vi "SIM_Drive_ODOM_BEGIN.vi"(8 "error in (no error)":errorcluster, 9 "Initial Pose":T3 {"ROTATION"."SIN" format="%13.4f"; "ROTATION"."COS" format="%13.4f"; "ROTATION"."VALUE" format="%13.4f"; "TRANSLATION"."Y" format="%14.3f"; "TRANSLATION"."X" format="%14.3f"}, 10 "Initial Gyro Angle":T2 {"SIN" format="%13.4f"; "COS" format="%13.4f"; "VALUE" format="%13.4f"}, 11 "Module Positions":T1[](array[typedef]) {"Angle"."SIN" format="%13.4f"; "Angle"."COS" format="%13.4f"; "Angle"."VALUE" format="%13.4f"}) -> (0 "error out":errorcluster)   [LabVIEW 2023]
uses:
  <vilib>/Rock Robotics/WPI/ThirdParty/JAS_Junk/TrajLib/TypeDef/ROTATION2D.ctl
  <vilib>/Rock Robotics/WPI/ThirdParty/JAS_Junk/TrajLib/TypeDef/POSE2D.ctl
  <vilib>/Rock Robotics/WPI/ThirdParty/JAS_Junk/TrajLib/TypeDef/TRANSLATION2D.ctl
  <vilib>/Rock Robotics/WPI/ThirdParty/JAS_Junk/TrajLib/Pose2d_getRotation.vi
  <vilib>/Rock Robotics/WPI/ThirdParty/JAS_Junk/TrajLib/Rotation2d_Minus.vi
  <vilib>/Rock Robotics/SystemInterfaces/NetworkCommunication/NetComm_UsageReport_report.vi
  <vilib>/Rock Robotics/WPI/ThirdParty/JAS_Junk/TrajLib/Rotation2d_UnaryMinus.vi
  <vilib>/Rock Robotics/WPI/ThirdParty/JAS_Junk/TrajLib/Rotation2d_RotateBy.vi
  <vilib>/Rock Robotics/WPI/ThirdParty/JAS_Junk/TrajLib/Rotation2d_CreateAngle.vi
  <vilib>/Rock Robotics/WPI/ThirdParty/JAS_Junk/TrajLib/Rotation2d_CreateXY.vi
  <vilib>/Rock Robotics/WPI/ThirdParty/JAS_Junk/TrajLib/Util_CalcDist.vi
  <vilib>/Rock Robotics/WPI/ThirdParty/JAS_Junk/TrajLib/Globals/Util_LibraryGlobals.vi
  SIM_Drive_Globals.vi
  <vilib>/Rock Robotics/WPI/ThirdParty/JAS_Junk/TrajLib/Trajectory_Library.lvlib
  <vilib>/Rock Robotics/WPI/ThirdParty/JAS_Junk/TrajLib/TypeDef/SWERVE_DRIVE_MODULE_POSITION.ctl
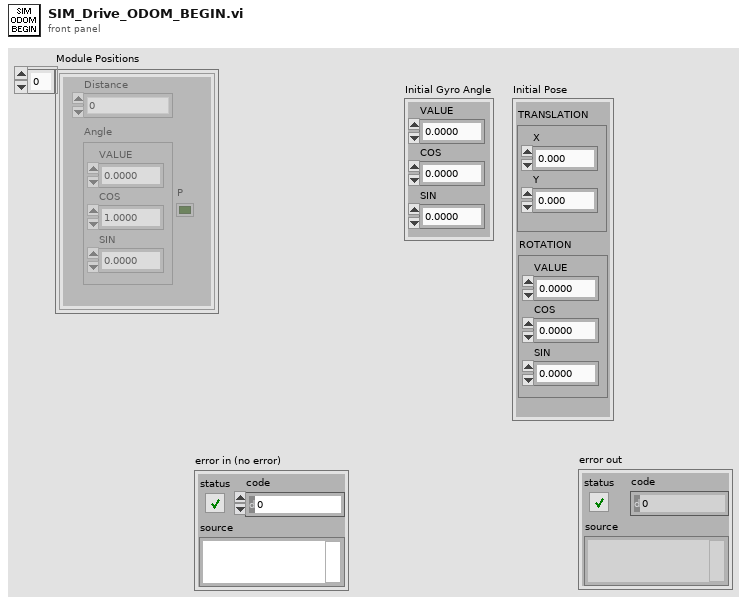
[diagram p1: front panel]
types:
  T1 = typedef "Trajectory_Library.lvlib/SWERVE_DRIVE_MODULE_POSITION.ctl" = cluster{"Distance":dbl, "Angle":T2, "P":bool}
  T2 = typedef "Trajectory_Library.lvlib/ROTATION2D.ctl" = cluster{"VALUE":dbl, "COS":dbl, "SIN":dbl}
  T3 = typedef "Trajectory_Library.lvlib/POSE2D.ctl" = cluster{"TRANSLATION":T4, "ROTATION":T2}
  T4 = typedef "Trajectory_Library.lvlib/TRANSLATION2D.ctl" = cluster{"X":dbl, "Y":dbl}
  T5 = typedef "Trajectory_Library.lvlib/SWERVE_DRIVE_ODOMETRY.ctl" = cluster{"POSE":T3, "GyroOffset":T2, "PreviousAngle":T2, "PrevModulePositions":T1[], "NumModules":i32}
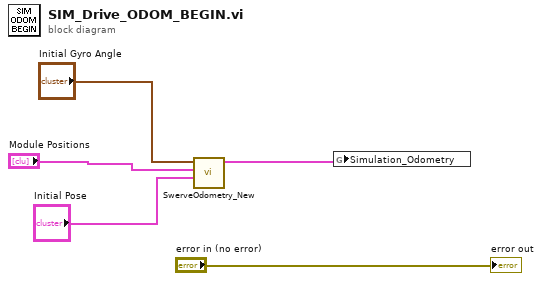
[diagram p0: block diagram]
diagram:
  n1 = call <vilib>:"SwerveOdometry_New.vi"("InitialPose"="Initial Pose", "Module Positions"="Module Positions", "gyroAngle"="Initial Gyro Angle") -> ("SWERVE_DRIVE_ODOMETRY"=w2:T5)  [unwired: 8 in]
  n2 = global write "SIM_Drive_Globals.vi" "Simulation_Odometry"(w2) -> ()
  "error out" <- "error in (no error)"
